vi "[SubVI]Incremental_ENC.vi"(4 "Left Reset":bool, 5 "Right Reset":bool, 6 "Left Motor ENC":T1, 7 "Right Motor ENC":T1) -> (0 "Left INC":i32, 1 "Right INC":i32, 2 "Left Motor ENC Out":T1, 3 "Right Motor ENC Out":T1)   [LabVIEW 2017]
uses:
  <vilib>/myRIO/Instrument Drivers/Onboard IO/Encoder/typedefs/Encoder Reference.ctl
  <vilib>/myRIO/Common/Instrument Driver Framework/Utilities/typedefs/myRIO Generic Hardware Reference.ctl
  <vilib>/myRIO/Common/Instrument Driver Framework/Utilities/typedefs/Hardware Version Enum.ctl
  <vilib>/myRIO/Common/Instrument Driver Framework/Utilities/typedefs/myRIO v1.0 Reference.ctl
  <vilib>/myRIO/Common/Instrument Driver Framework/Utilities/typedefs/Generic FPGA Reference.ctl
  <vilib>/myRIO/Common/Instrument Driver Framework/myRIO v1.0/Encoder/typedefs/Encoder Channels Enum.ctl
  <vilib>/Utility/error.llb/Error Cluster From Error Code.vi
  <vilib>/myRIO/Common/Instrument Driver Framework/myRIO v1.0/Encoder/vis/myRIO v1.0 Read Encoder.vi
  <vilib>/myRIO/Instrument Drivers/Onboard IO/Encoder/Encoder.lvlib
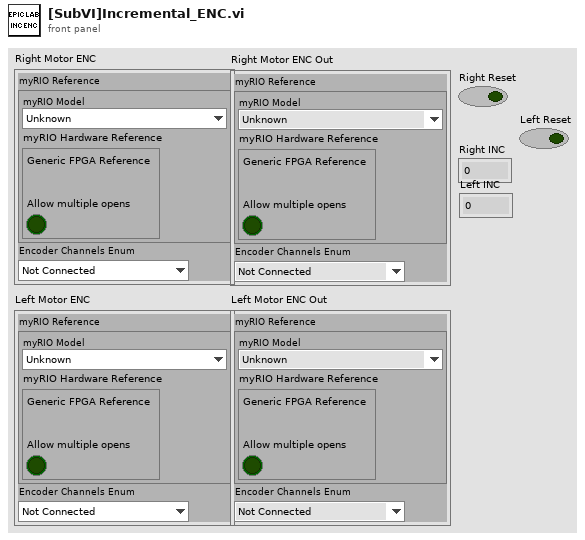
[diagram p1: front panel]
types:
  T1 = typedef "Encoder.lvlib/Encoder Reference.ctl" = cluster{"myRIO Reference":T2, "Encoder Channels Enum":T6}
  T2 = typedef "myRIO Generic Hardware Reference.ctl" = cluster{"myRIO Model":T3, "myRIO Hardware Reference":T4}
  T3 = typedef "Hardware Version Enum.ctl" = enum16{"Unknown", "myRIO-1900", "myRIO-1950", "roboRIO", "NI ELVIS RIO CM"}
  T4 = typedef "myRIO v1.0 Reference.ctl" = cluster{"Generic FPGA Reference":T5, "Allow multiple opens":bool}
  T5 = typedef "Generic FPGA Reference.ctl" = refnum<k20>
  T6 = typedef "Encoder Channels Enum.ctl" = enum16{"Not Connected", "C/ENC0", "C/ENC1", "A/ENC", "B/ENC", "DIO/ENC0", "DIO/ENC1", "DIO/ENC2", "DIO/ENC3", "DIO/ENC4"}
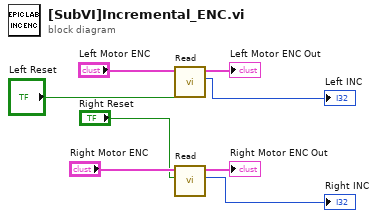
[diagram p0: block diagram]
diagram:
  n1 = call <vilib>:"Read.vi"("Reset Counter"="Left Reset", "Encoder Ref In"="Left Motor ENC") -> ("Counter Value"=→"Left INC":i32, "Encoder Ref Out"=→"Left Motor ENC Out":T1)  [unwired: 5 in, 3 out]
  n2 = call <vilib>:"Read.vi"("Reset Counter"="Right Reset", "Encoder Ref In"="Right Motor ENC") -> ("Counter Value"=→"Right INC":i32, "Encoder Ref Out"=→"Right Motor ENC Out":T1)  [unwired: 5 in, 3 out]
